vi "校准数据写入配置文件.vi"(8 "error in (no error)":errorcluster caption="错误输入（无错误）") -> (0 "错误输出":errorcluster)   [LabVIEW 2016, in "斯坦道CODMn新电路板.lvlib"]
uses:
  <vilib>/Utility/xml.llb/Write to XML File(string).vi
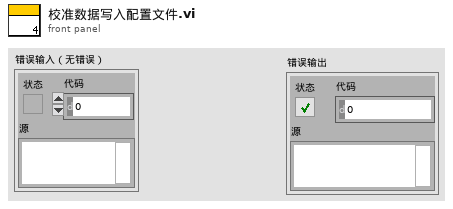
[diagram p1: front panel]
types:
  T1 = cluster{"标液浓度1":dbl, "测量吸光度1":dbl, "样品1启用":bool, "标液浓度2":dbl, "测量吸光度2":dbl, "样品2启用":bool, "标液浓度3":dbl, "测量吸光度3":dbl, "样品3启用":bool, "标液浓度4":dbl, "测量吸光度4":dbl, "样品4启用":bool, "标液浓度5":dbl, "测量吸光度5":dbl, "样品5启用":bool, "模型":enum32{"线性", "多项式"}, "精度":dbl, "XY图":cluster{"X Values":dbl[], "Y Values":dbl[]}[], "拟合公式":string, "r^2":dbl, "标样一校准时间":timestamp, "标样二校准时间":timestamp, "标样三校准时间":timestamp, "标样四校准时间":timestamp, "标样五校准时间":timestamp, "二次方程":cluster{"c":dbl, "x":dbl, "x^2":dbl}, "标定时间":timestamp}[][]
  T2 = cluster{"CODMn曲线模型":cluster{"标液浓度1":dbl, "测量吸光度1":dbl, "样品1启用":bool, "标液浓度2":dbl, "测量吸光度2":dbl, "样品2启用":bool, "标液浓度3":dbl, "测量吸光度3":dbl, "样品3启用":bool, "标液浓度4":dbl, "测量吸光度4":dbl, "样品4启用":bool, "标液浓度5":dbl, "测量吸光度5":dbl, "样品5启用":bool, "模型":enum32{"线性", "多项式"}, "精度":dbl, "XY图":cluster{"X Values":dbl[], "Y Values":dbl[]}[], "拟合公式":string, "r^2":dbl, "标样一校准时间":timestamp, "标样二校准时间":timestamp, "标样三校准时间":timestamp, "标样四校准时间":timestamp, "标样五校准时间":timestamp, "二次方程":cluster{"c":dbl, "x":dbl, "x^2":dbl}, "标定时间":timestamp}[][]}
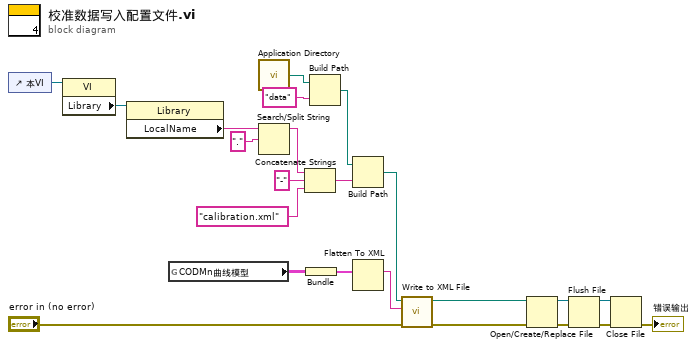
[diagram p0: block diagram]
diagram:
  n1 = control-ref of="本VI"() -> (w10:refnum<vi>)
  n2 = property class="VI"(reference=w10) -> ("Library"=w11:refnum<vi>)  [unwired: 1 in, 2 out]
  n3 = property class="Library"(reference=w11) -> ("LocalName"=w8:string)  [unwired: 1 in, 2 out]
  n4 = global read "校准数据全局变量.vi" "CODMn曲线模型"() -> (w12:T1)
  n5 = call <vilib>:"Application Directory.vi"() -> ("Application Directory"=w15:path)
  n6 = Search/Split String(string=w8, search string/char (-)="." ("搜索字符串/字符(-)")) -> (substring before match=w6:string)  [unwired: 1 in, 2 out]
  n7 = Concatenate Strings(w6, "-" ("字符串"), "calibration.xml" ("名称或相对路径")) -> (w3:string)
  n8 = Bundle("CODMn曲线模型"=w12) -> (w1:T2)  [unwired: 1 in]
  n9 = Build Path(base path=w15, name or relative path="data" ("名称或相对路径")) -> (appended path=w9:path)
  n10 = Build Path(base path=w9, name or relative path=w3) -> (appended path=w2:path)
  n11 = Flatten To XML(anything=w1) -> (xml string=w23:string)
  n12 = call-poly <vilib>:"Write to XML File.vi"("error in (no error)"="error in (no error)", "XML Input"=w23, "XML File Path"=w2) -> ("error out"=w18:errorcluster, "XML File Path(duplicate)"=w17:path)  [unwired: 6 in, 1 out]
  n13 = Open/Create/Replace File(file path (use dialog)=w17, error in=w18) -> (refnum out=w21:refnum<file>, error out=w22:errorcluster)  [unwired: 4 in, 1 out]
  n14 = Flush File(refnum=w21, error in=w22) -> (refnum out=w20:refnum<file>, error out=w19:errorcluster)
  n15 = Close File(refnum=w20, error in=w19) -> (error out=→"错误输出":errorcluster)  [unwired: 1 out]
